vi "Mouse Left Click.vi"   [LabVIEW 2015]
uses:
  USER32.DLL
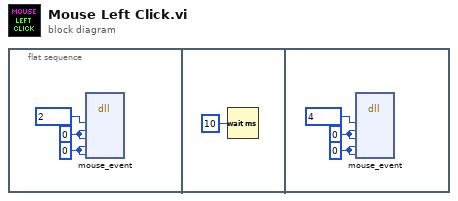
[diagram p0: block diagram]
diagram:
  n1 = flat-sequence {
    frame #0 {
      w3 = 0 ("dwExtraInfo")
      w2 = u32 0 ("dwExtraInfo")
      n2 = dll-call lib="user32.dll" fn="mouse_event" label="mouseeventf_leftdown"("dwFlags"=2, "dx"=w3, "dy"=w3, "dwData"=w2, "dwExtraInfo"=w2) -> ()  [unwired: 9 in, 2 out]
    }
    frame #1 {
      n3 = Wait (ms)(milliseconds to wait=u32 10) -> ()  [unwired: 1 out]
    }
    frame #2 {
      w7 = 0 ("dwExtraInfo")
      w6 = u32 0 ("dwExtraInfo")
      n4 = dll-call lib="user32.dll" fn="mouse_event" label="mouseeventf_leftup"("dwFlags"=4, "dx"=w7, "dy"=w7, "dwData"=w6, "dwExtraInfo"=w6) -> ()  [unwired: 9 in, 2 out]
    }
  }
